vi "REWORK_prepare_diagnostics_record_for_buffer.vi"(7 "message_type":T2, 8 "to":string, 9 "from":string, 10 "message":string) -> (3 "record":T1)   [LabVIEW 2019]
uses:
  _misc/DIAGNOSTICS_message_type.ctl
  FGV/DIAGNOSTICS_message_history_buffer/REWORK_DIAGNOSTICS_message_history_buffer_all_info.ctl
  _misc/AULocalize/SubVIs/Get Localized Phrase Compact Interface 0D.vi
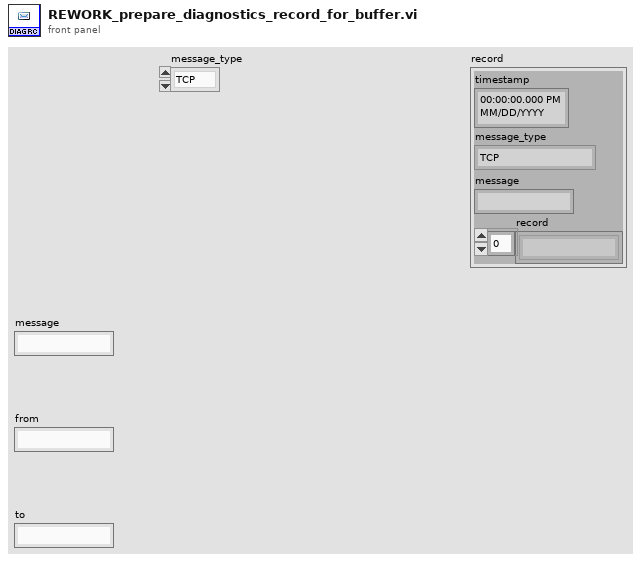
[diagram p1: front panel]
types:
  T1 = typedef "REWORK_DIAGNOSTICS_message_history_buffer_all_info.ctl" = cluster{"timestamp":timestamp, "message_type":T2, "message":string, "record":string[]}
  T2 = typedef "DIAGNOSTICS_message_type.ctl" = enum16{"TCP", "SQL"}
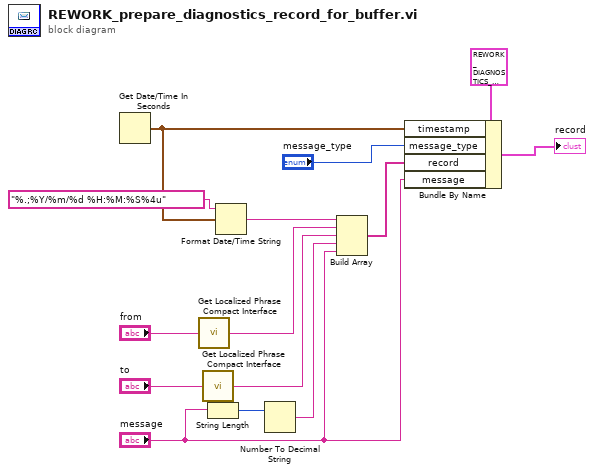
[diagram p0: block diagram]
diagram:
  n1 = Get Date/Time In Seconds() -> (seconds since 1Jan1904=w6:timestamp)
  n2 = call-poly "Get Localized Phrase Compact Interface.vi"("Key"="from") -> ("Translated Phrase"=w2:string)
  n3 = call-poly "Get Localized Phrase Compact Interface.vi"("Key"="to") -> ("Translated Phrase"=w1:string)
  n4 = String Length(string="message") -> (length=w5:i32)
  n5 = Format Date/Time String(time format string (%c)="%.;%Y/%m/%d %H:%M:%S%4u", seconds (now)=w6) -> (date/time string=w11:string)  [unwired: 1 in]
  n6 = Number To Decimal String(number=w5) -> (decimal integer string=w4:string)  [unwired: 1 in]
  n7 = Build Array(w11, w2, w1, w4, "message") -> (w12:string[])
  n8 = Bundle By Name(cluster=T1 {"timestamp"=timestamp(0 s since 1904-01-01), "message_type"=enum."TCP", "message"="", "record"=[]} ("Cluster"), "timestamp"=w6, "message_type"="message_type", "record"=w12, "message"="message") -> (→"record":T1)
